vi "createChannel.vi"(8 "error in (no error)":errorcluster, 11 "HamegHMPSupply in":refnum<class "HamegHMPSupply.lvclass">) -> (0 "error out":errorcluster, 3 "HamegHMPSupply out":refnum<class "HamegHMPSupply.lvclass">)   [LabVIEW 2009, in "Hardware.lvlib" / "Channels.lvlib" / "HamegHMPSupply.lvclass"]
doc: "Abstract Method.\n\nCreates an analog output channel by reserving hardware resources needed by the output. This vi sets a name for the channel, and via its implementation classes (such as niDAQmxAO etc) reserves the physical channel on the output device."
uses:
  HamegHMPSupply.lvclass
  AnalogOutput.lvclass
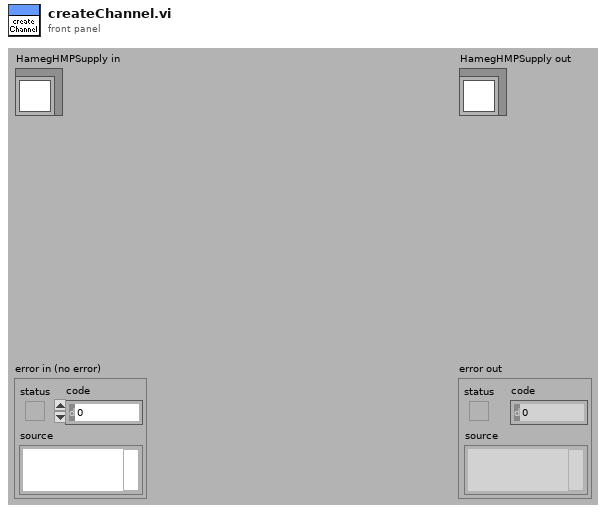
[diagram p1: front panel]
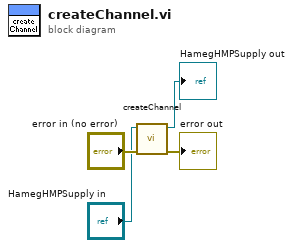
[diagram p0: block diagram]
diagram:
  n1 = call-parent "createChannel.vi"("error in (no error)"="error in (no error)", "AnalogOutput in"="HamegHMPSupply in") -> ("error out"=→"error out":errorcluster, "AnalogOutput out"=→"HamegHMPSupply out":refnum<class "HamegHMPSupply.lvclass">)  [unwired: 8 in]
